vi "AxisCutter(Simtools).vi"(0 "수신":string) -> (1 "Axis":string, 2 "L":i32, 3 "R":i32, 4 "M":i32)   [LabVIEW 2013]
panel:
  out "END":string
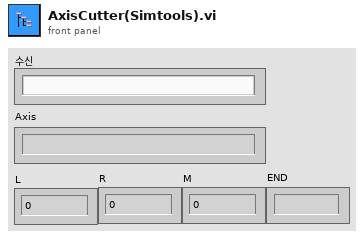
[diagram p1: front panel]
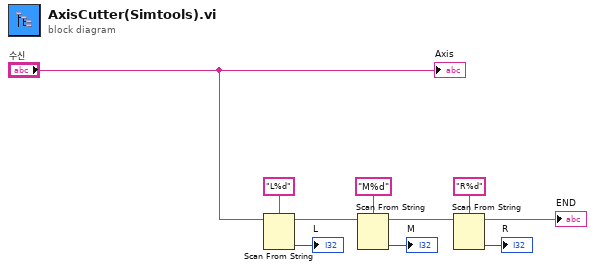
[diagram p0: block diagram]
diagram:
  n1 = Scan From String(format string="L%d" ("포맷 문자열"), input string="수신") -> (remaining string=w4:string, output 1=→"L":i32)  [unwired: 3 in, 2 out]
  n2 = Scan From String(format string="M%d" ("포맷 문자열"), input string=w4) -> (remaining string=w3:string, output 1=→"M":i32)  [unwired: 3 in, 2 out]
  n3 = Scan From String(format string="R%d" ("포맷 문자열"), input string=w3) -> (remaining string=→"END":string, output 1=→"R":i32)  [unwired: 3 in, 2 out]
  "Axis" <- "수신"
